vi "Database Command Get Parameters Ref.vi"(8 "error in (no error)":errorcluster caption="错误输入（无错误）", 11 "Database Command 输入":refnum<class "Database Command.lvclass"> caption="DNL_LabVIEW Object in") -> (0 "error out":errorcluster caption="错误输出", 3 "Database Command 输出":refnum<class "Database Command.lvclass"> caption="DNL_LabVIEW Object out")   [LabVIEW 2011, in "Database Command.lvclass"]
uses:
  Database Command.lvclass
  Database Command.lvclass/Database Command.ctl
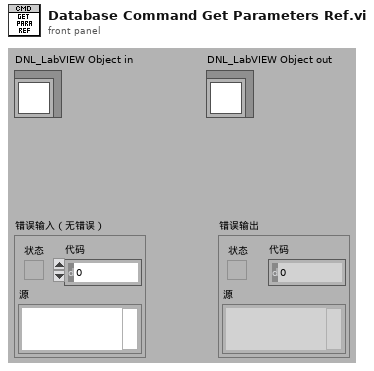
[diagram p1: front panel]
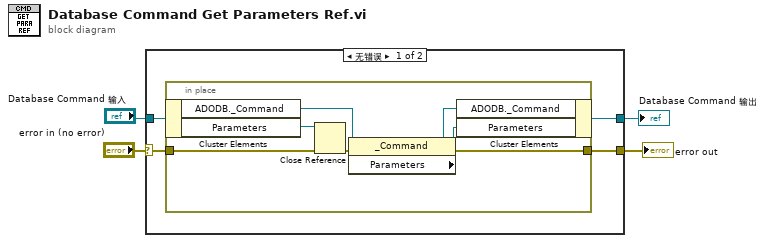
[diagram p0: block diagram]
diagram:
  n1 = case shown="无错误" "error in (no error)" {
    selector: "error in (no error)" -> [w7 w17]
    tunnel: [w6 w17] -> w3
    tunnel: [w5 w16] -> w1
    tunnel: "Database Command 输入" -> [w8 w16]
    frame No Error {
      n2 = in-place {
        in-place-border: w7 -> [w11]
        in-place-border: [w12] -> w6
        n3 = in-place-cluster #1(w8) -> ("ADODB._Command"=w15:refnum<k7>, "Parameters"=w9:refnum<k7>)
        n4 = Close Reference(reference=w9, error in (no error)=w11) -> (error out=w10:errorcluster)
        n5 = property class="_Command"(reference=w15, error in=w10) -> (reference out=w13:refnum<k7>, error out=w12:errorcluster, "Parameters"=w14:refnum<k7>)
        n6 = in-place-cluster #1("ADODB._Command"=w13, "Parameters"=w14) -> (w5:refnum<class "Database Command.lvclass">)
      }
    }
    frame Error {
    }
  }
  "error out" <- w3
  "Database Command 输出" <- w1
